vi "niRFUtil MASMT Resample (constant to constant) (multi-channel, CDB).vi"(5 "anti-aliasing?":bool=TRUE, 6 "FIR filter specifications":T1={"alias rejection (dB)"=120.0, "normalized bandwidth"=0.4536}, 7 "reset?":bool, 8 "error in (no error)":errorcluster, 9 "dt":dbl=1.0, 10 "delay":dbl, 11 "X":cdb[][](array[numeric])) -> (0 "error out":errorcluster, 2 "t0":dbl, 3 "Y":cdb[][](array[numeric]) format="%#.6g")   [LabVIEW 2015, in "niRFUtil.lvlib"]
doc: "Resamples input signal <B>X</B> according to <B>delay</B> and <B>dt</B> using an FIR filter implementation."
uses:
  niRFUtil.lvlib
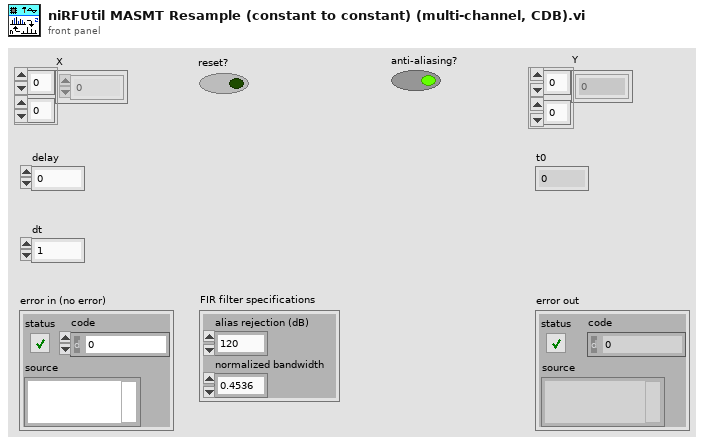
[diagram p1: front panel]
types:
  T1 = cluster{"alias rejection (dB)":dbl, "normalized bandwidth":dbl}
  T2 = cluster{"new sample period":dbl, "first point location":dbl, "timing jitter":i32}
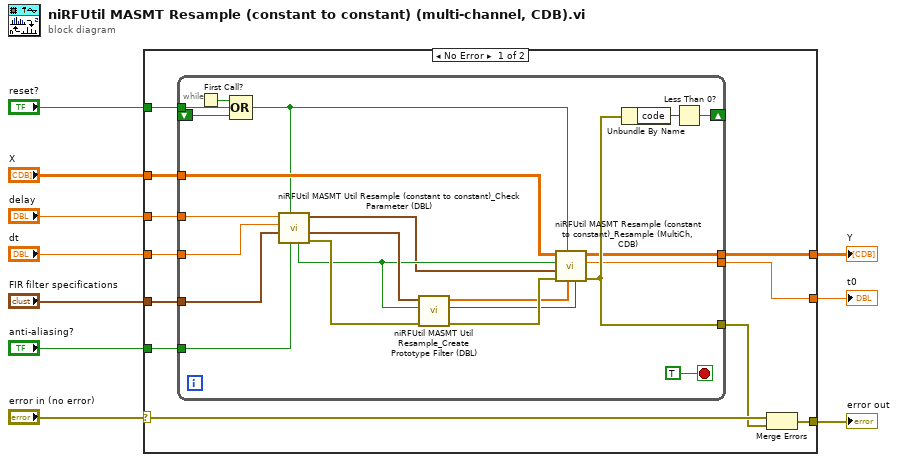
[diagram p0: block diagram]
diagram:
  n1 = case shown="No Error" "error in (no error)" {
    selector: "error in (no error)" -> [w14 w44]
    tunnel: "FIR filter specifications" -> [w15 _]
    tunnel: "dt" -> [w11 _]
    tunnel: "delay" -> [w17 _]
    tunnel: "reset?" -> [w16 _]
    tunnel: "X" -> [w21 _]
    tunnel: "anti-aliasing?" -> [w20 _]
    tunnel: [w12 w44] -> w1
    tunnel: [w19 _] -> w2
    tunnel: [w18 _] -> w3
    frame No Error {
      n2 = while {
        tunnel: w17 -> [w36]
        tunnel: w16 -> [w40]
        tunnel: [w23] -> w19
        tunnel: [w22] -> w18
        tunnel: w11 -> [w35]
        tunnel: w21 -> [w31]
        tunnel: w20 -> [w33]
        tunnel: [w24] -> w13
        shift-right: [w41] -> _
        shift-left: _ -> [w38]
        tunnel: w15 -> [w37]
        stop <- TRUE stop-if-true
        n3 = First Call?() -> (First Call?: T/F=w39:bool)
        n4 = Compound Arithmetic op=OR(w39, w40, w38) -> (w29:bool)
        n5 = call "niRFUtil MASMT Util Resample (constant to constant)_Check Parameter (DBL).vi"("anti-aliasing in"=w33, "reset?"=w29, "FIR filter specifications in"=w37, "dt"=w35, "delay"=w36) -> ("error out"=w34:errorcluster, "FIR filter specifications out"=w32:T1, "config"=w28:T2, "anti-aliasing out"=w30:bool)  [unwired: 3 in]
        n6 = call "niRFUtil MASMT Util Resample_Create Prototype Filter (DBL).vi"("error in (no error)"=w34, "anti-aliasing?"=w30, "FIR filter specifications"=w32) -> ("error out"=w27:errorcluster, "decimation factor"=w25:i32, "Coefficients"=w26:dbl[])  [unwired: 6 in]
        n7 = call "niRFUtil MASMT Resample (constant to constant)_Resample (MultiCh, CDB).vi"("max decimation"=w25, "Resample FIR"=w26, "reset?"=w29, "error in (no error)"=w27, "config"=w28, "anti-aliasing?"=w30, "X"=w31) -> ("error out"=w24:errorcluster, "t0"=w23:dbl, "Y"=w22:cdb[][])  [unwired: 2 in]
        n8 = Unbundle By Name(w24) -> ("code"=w42:i32)
        n9 = Less Than 0?(x=w42) -> (x < 0?=w41:bool)
      }
      n10 = Merge Errors(w14, w13) -> (w12:errorcluster)
    }
    frame Error {
    }
  }
  "error out" <- w1
  "Y" <- w3
  "t0" <- w2
